vi "Get Handlers.vi"(8 "error in":errorcluster) -> (0 "error out":errorcluster, 3 "Handlers":refnum<class "Handler.lvclass">[](array[class]))   [LabVIEW 2024, in "hse-logger.lvlib"]
doc: "Returns a Handler from the logger specified by name.\nIf name was not found, returns a basis handler without functionality and raise an error \"510802 - Handler name not found\".\n\n____\nHAMPEL SOFTWARE ENGINEERING v2.2.2 (2025-01-16 15:41)"
uses:
  <vilib>/Hampel Software Engineering/HSE Logger/hse-logger.lvlib
  <vilib>/Hampel Software Engineering/HSE Logger/Handler/Handler.lvclass
  <vilib>/Hampel Software Engineering/HSE Logger/FGV Actions.ctl
  <vilib>/Hampel Software Engineering/HSE Logger/Logger/Logger.lvclass
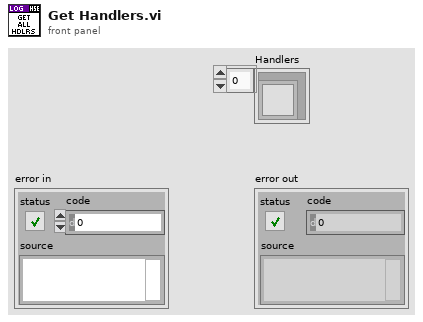
[diagram p1: front panel]
types:
  T1 = typedef "hse-logger.lvlib/FGV Actions.ctl" = enum16{"Set", "Get"}
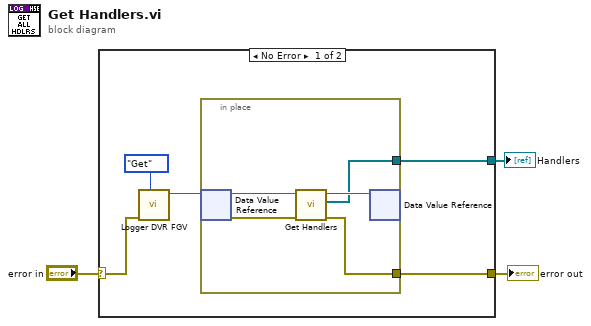
[diagram p0: block diagram]
diagram:
  n1 = case shown="No Error" "error in" {
    selector: "error in" -> [w8 w14]
    tunnel: [w7 w14] -> w2
    tunnel: [w5 _] -> w1
    frame No Error {
      n2 = call <vilib>:"Logger DVR FGV.vi"("FGV Actions"=FGV_Actions."Get", "error in"=w8) -> ("Logger DVR"=w6:refnum<data-value>)  [unwired: 8 in, 1 out]
      n3 = in-place {
        in-place-border: [w9] -> w5
        in-place-border: [w13] -> w7
        n4 = in-place-dvr #1(w6) -> (w11:refnum<class "Logger.lvclass">, w12:errorcluster)
        n5 = call-dynamic "Get Handlers.vi"("error in"=w12, "Logger in"=w11) -> ("error out"=w13:errorcluster, "Handlers"=w9:refnum<class "Handler.lvclass">[], "Logger out"=w10:refnum<class "Logger.lvclass">)  [unwired: 7 in]
        n6 = in-place-dvr #1(w10) -> ()  [unwired: 2 out]
      }
    }
    frame Error {
    }
  }
  "error out" <- w2
  "Handlers" <- w1
